vi "Initialize.vi"(8 "error in":errorcluster, 11 "CRD Subject in":refnum<class "CRD Subject.lvclass">) -> (0 "error out":errorcluster, 2 "DVR":refnum<data-value>, 3 "CRD Subject out":refnum<class "CRD Subject.lvclass">)   [LabVIEW 2015, in "CRD Subject.lvclass"]
doc: "Provides a reference for the CRD Data object."
uses:
  CRD Subject.lvclass
  Reusable/Data/Data.lvclass
  Reusable/CRDS/Data/Main/CRDS Data.lvclass
  Reusable/Observer/Data Subject.lvclass/Data Subject.ctl
  Reusable/Observer/Data Subject.lvclass
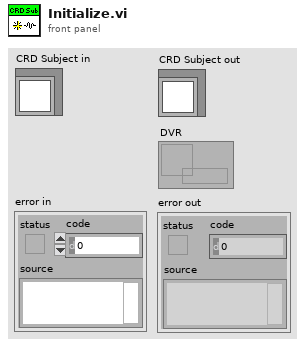
[diagram p1: front panel]
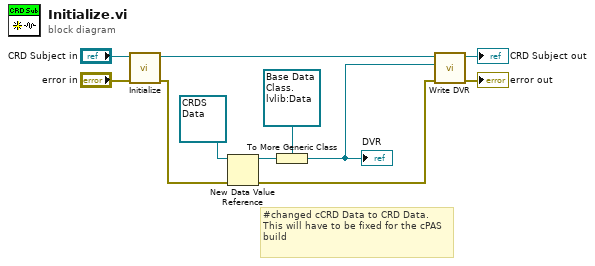
[diagram p0: block diagram]
diagram:
  # "#changed cCRD Data to CRD Data.  This will have to be fixed for the cPAS build"
  n1 = call-parent "Initialize.vi"("error in"="error in", "Data Subject in"="CRD Subject in") -> ("error out"=w6:errorcluster, "Data Subject out"=w1:refnum<class "CRD Subject.lvclass">)  [unwired: 7 in, 1 out]
  n2 = New Data Value Reference(data value=refnum<class "CRDS Data.lvclass"> refnum ("CRDS"), error in=w6) -> (data value reference=w8:refnum<data-value>, error out=w7:errorcluster)
  n3 = To More Generic Class(target class=refnum<data-value> refnum ("data value reference"), reference=w8) -> (generic class reference=w3:refnum<data-value>)
  "DVR" <- w3
  n4 = call "Write DVR.vi"("error in"=w7, "DVR"=w3, "Data Subject in"=w1) -> ("error out"=→"error out":errorcluster, "Data Subject out"=→"CRD Subject out":refnum<class "CRD Subject.lvclass">)  [unwired: 7 in]
